vi "Set Port.vi"(8 "error in (no error)":errorcluster, 10 "Port":refnum<k21>, 11 "MPU in":refnum<class "MPU.lvclass">) -> (0 "error out":errorcluster, 3 "MPU out":refnum<class "MPU.lvclass">)   [LabVIEW 2018]
uses:
  MPU.lvclass
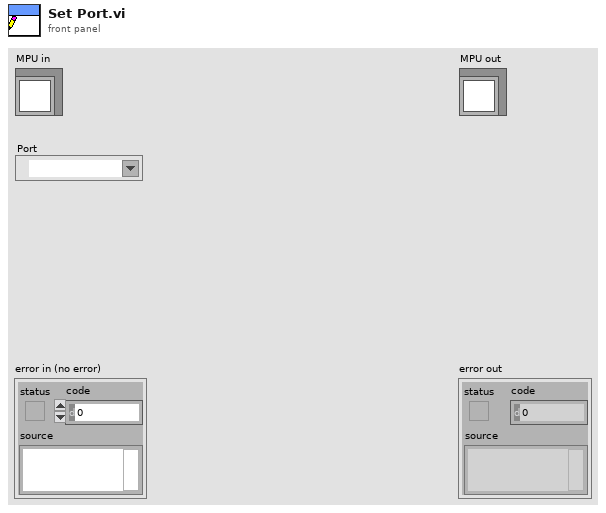
[diagram p1: front panel]
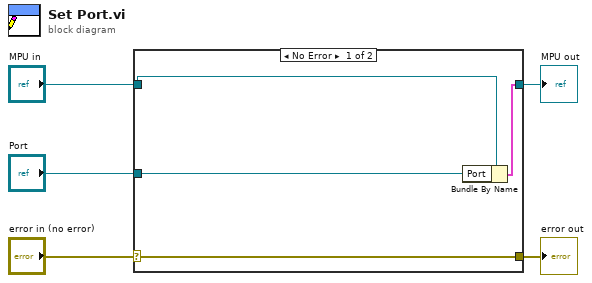
[diagram p0: block diagram]
diagram:
  n1 = case shown="No Error" "error in (no error)" {
    selector: "error in (no error)" -> [w9 w10]
    tunnel: [w9 w10] -> w4
    tunnel: [w7 w11] -> w2
    tunnel: "MPU in" -> [w8 w11]
    tunnel: "Port" -> [w6 _]
    frame No Error {
      n2 = Bundle By Name(cluster=w8, "Port"=w6) -> (w7:cluster{})
    }
    frame Error {
    }
  }
  "error out" <- w4
  "MPU out" <- w2
